vi "testpsp.vi"() -> ()   [LabVIEW 2013, in "testvarlib.lvlib"]
uses:
  testvarlib.lvlib
  execution/Scan Engine runtime.lvclass
  <vilib>/NI/Tag Bus Module Framework/channel/channel classification.ctl
  configuration/url prefix.ctl
  <vilib>/NI/Tag Bus/tag/Data Type.ctl
  configuration/Scan Engine configuration.lvclass
  configuration/Scan Engine configuration.lvclass/Scan Engine configuration.ctl
  <vilib>/NI/Tag Bus/table/data polymorphs/write one/write Double.vi
  <vilib>/NI/Tag Bus/table/data polymorphs/read one/read Double.vi
  configuration/Write discover channels.vi
  configuration/Write configure scan engine.vi
  <vilib>/NI/Tag Bus/table/data table.lvlib
  <vilib>/NI/Tag Bus/tag/tag descriptor.lvclass
  <vilib>/NI/Tag Bus Module Framework/channel/TBM channel.lvclass
panel:
  in  "testvarin":dbl
  out "testvarout":dbl
  in  "testvaroutTB":dbl
  in  "stop":bool
  out "ok":bool
  out "testvarinTB":dbl
  out "final error":errorcluster
  out "output error":errorcluster
  out "input error":errorcluster
  out "init error":errorcluster
  out "correct execution settings":bool
  out "serialization problem":errorcluster
  out "invalid configuration":errorcluster
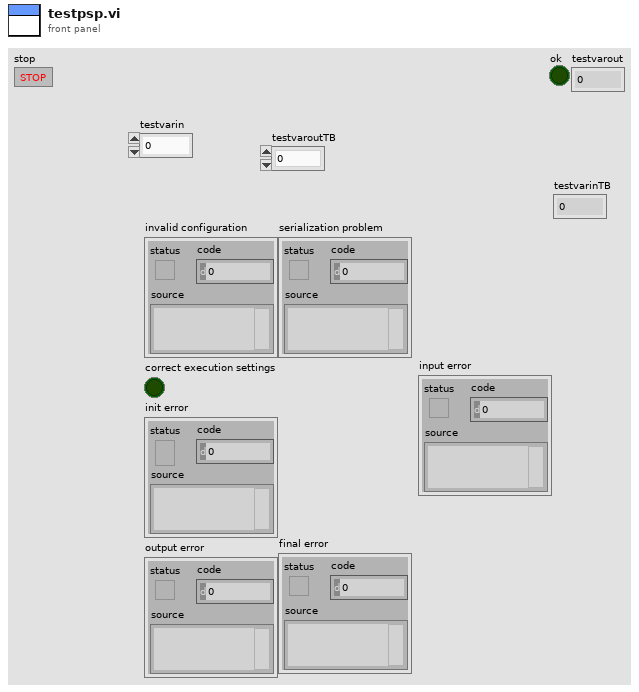
[diagram p1: front panel]
types:
  T1 = typedef "TBM channel.lvclass/channel classification.ctl" = enum16{"input data", "output data", "processing parameter", "processing result"}
  T2 = typedef "tag bus.lvlib/tag descriptor.lvclass/Data Type.ctl" = enum16{"Double", "Single", "I64", "I32", "I16", "I8", "U64", "U32", "U16", "U8", "Boolean", "String", "Array of Double", "Array of Single", "Array of I64", "Array of I32", "Array of I16", "Array of I8", "Array of U64", "Array of U32", "Array of U16", "Array of U8", "Array of Boolean", "Array of String"}
  T3 = typedef "Scan Engine configuration.lvclass/url prefix.ctl" = enum32{"ni.var.io://", "ni.var.psp://"}
  T4 = typedef "TBM channel.lvclass/data tables.ctl" = cluster{"input data":T5, "processing parameter":T5, "processing result":T5, "output data":T5}
  T5 = typedef "tag bus.lvlib/dictionary table pair.ctl" = cluster{"data dictionary":refnum<class "data dictionary.lvclass">, "data table":T6}
  T6 = typedef "tag bus.lvlib/data table.lvlib/data table.ctl" = cluster{"Double":dbl[], "Single":sgl[], "I64":i64[], "I32":i32[], "I16":i16[], "I8":i8[], "U64":u64[], "U32":u32[], "U16":u16[], "U8":u8[], "Boolean":bool[], "String":string[], "Array of Double":cluster{"DBL Array":dbl[]}[], "Array of Single":cluster{"SGL Array":sgl[]}[], "Array of I64":cluster{"I64 Array":i64[]}[], "Array of I32":cluster{"I32 Array":i32[]}[], "Array of I16":cluster{"I16 Array":i16[]}[], "Array of I8":cluster{"I8 Array":i8[]}[], "Array of U64":cluster{"U64 Array":u64[]}[], "Array of U32":cluster{"U32 Array":u32[]}[], "Array of U16":cluster{"U16 Array":u16[]}[], "Array of U8":cluster{"U8 Array":u8[]}[], "Array of Boolean":cluster{"Boolean Array":bool[]}[], "Array of String":cluster{"String Array":string[]}[]}
  T7 = typedef "TBM module execution interface.lvclass/execution settings.ctl" = cluster{"reads inputs":bool, "processes data":bool, "writes outputs":bool}
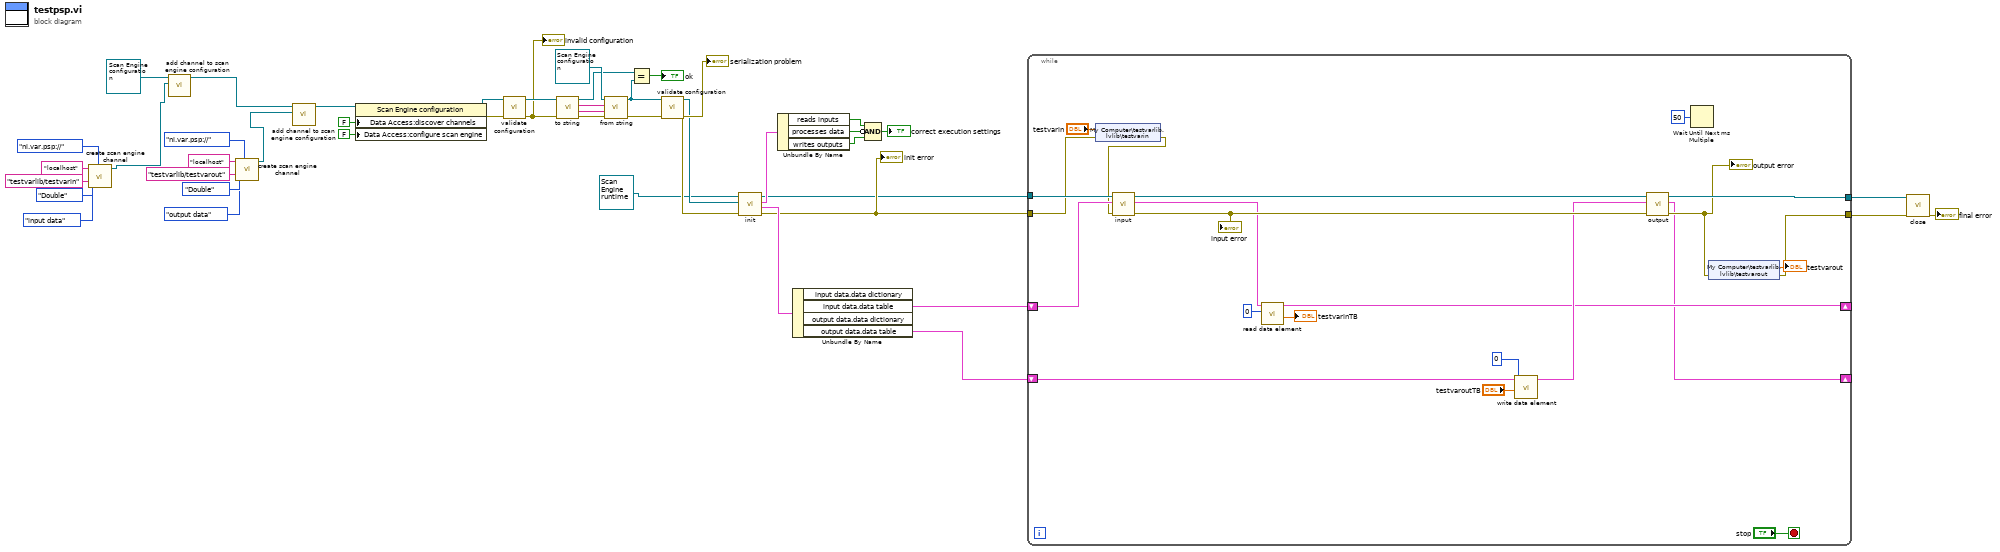
[diagram p0: block diagram]
diagram:
  n1 = call "create scan engine channel.vi"("URL"=url_prefix."ni.var.psp://", "channel classification"=channel_classification."input data", "data type"=Data_Type."Double", "variable name"="testvarlib/testvarin", "hostname"="localhost") -> ("channel"=w8:refnum<class "TBM channel.lvclass">)  [unwired: 6 in]
  n2 = call "add channel to scan engine configuration.vi"("channel"=w8, "Scan Engine configuration in"=refnum<class "Scan Engine configuration.lvclass"> refnum ("Scan Engine configuration")) -> ("Scan Engine configuration out"=w19:refnum<class "Scan Engine configuration.lvclass">)  [unwired: 8 in, 1 out]
  n3 = call "create scan engine channel.vi"("URL"=url_prefix."ni.var.psp://", "channel classification"=channel_classification."output data", "data type"=Data_Type."Double", "variable name"="testvarlib/testvarout", "hostname"="localhost") -> ("channel"=w7:refnum<class "TBM channel.lvclass">)  [unwired: 6 in]
  n4 = call "add channel to scan engine configuration.vi"("channel"=w7, "Scan Engine configuration in"=w19) -> ("Scan Engine configuration out"=w20:refnum<class "Scan Engine configuration.lvclass">)  [unwired: 8 in, 1 out]
  n5 = property class="Scan Engine configuration"(reference=w20, "Data Access:discover channels"=FALSE ("discover channels"), "Data Access:configure scan engine"=FALSE ("configure scan engine")) -> (reference out=w26:refnum<class "Scan Engine configuration.lvclass">, error out=w25:errorcluster)  [unwired: 1 in]
  n6 = call-dynamic "validate configuration.vi"("error in"=w25, "Scan Engine configuration in"=w26) -> ("error out"=w44:errorcluster, "Scan Engine configuration out"=w45:refnum<class "Scan Engine configuration.lvclass">)  [unwired: 8 in]
  "invalid configuration" <- w44
  n7 = call-dynamic "to string.vi"("error in"=w44, "Scan Engine configuration in"=w45) -> ("error out"=w41:errorcluster, "data"=w42:string, "version"=w43:string, "Scan Engine configuration out"=w4:refnum<class "Scan Engine configuration.lvclass">)  [unwired: 6 in]
  n8 = call-dynamic "from string.vi"("error in"=w41, "data"=w42, "version"=w43, "Scan Engine configuration in"=refnum<class "Scan Engine configuration.lvclass"> refnum ("Scan Engine configuration")) -> ("error out"=w40:errorcluster, "Scan Engine configuration out"=w3:refnum<class "Scan Engine configuration.lvclass">)  [unwired: 6 in]
  n9 = Equal?(x=w4, y=w3) -> (x = y?=→"ok":bool)
  n10 = call-dynamic "validate configuration.vi"("error in"=w40, "Scan Engine configuration in"=w3) -> ("error out"=w22:errorcluster, "Scan Engine configuration out"=w21:refnum<class "Scan Engine configuration.lvclass">)  [unwired: 8 in]
  "serialization problem" <- w22
  n11 = call-dynamic "init.vi"("error in"=w22, "TBM module configuration in"=w21, "Scan Engine runtime in"=refnum<class "Scan Engine runtime.lvclass"> refnum ("Scan Engine runtime")) -> ("error out"=w33:errorcluster, "data allocations"=w34:T4, "execution settings"=w39:T7, "Scan Engine runtime out"=w31:refnum<class "Scan Engine runtime.lvclass">)  [unwired: 5 in]
  "init error" <- w33
  n12 = Unbundle By Name(w39) -> ("reads inputs"=w36:bool, "processes data"=w38:bool, "writes outputs"=w37:bool)
  n13 = Unbundle By Name(w34) -> ("input data.data table"=w32:T6, "output data.data table"=w30:T6)  [unwired: 2 out]
  n14 = Compound Arithmetic op=AND(w36, invert w38, w37) -> (→"correct execution settings":bool)
  n15 = while {
    tunnel: w33 -> [w53]
    tunnel: w31 -> [w66]
    tunnel: [w61] -> w29
    tunnel: [w50] -> w28
    shift-right: [w47] -> _
    shift-left: w32 -> [w67]
    shift-right: [w46] -> _
    shift-left: w30 -> [w65]
    stop <- "stop" stop-if-true
    n16 = shared-variable "My Computer\\testvarlib.lvlib\\testvarin"("testvarin", error in=w53) -> (error out=w52:errorcluster)
    n17 = call-dynamic "input.vi"("error in"=w52, "data table in"=w67, "Scan Engine runtime in"=w66) -> ("error out"=w64:errorcluster, "data table out"=w60:T6, "Scan Engine runtime out"=w63:refnum<class "Scan Engine runtime.lvclass">)  [unwired: 6 in]
    "input error" <- w64
    n18 = call-poly <vilib>:"read data element.vi"("index"=0, "data table in"=w60) -> ("value"=→"testvarinTB":dbl, "data table out"=w47:T6)  [unwired: 8 in]
    n19 = call-poly <vilib>:"write data element.vi"("value"="testvaroutTB", "index"=0, "data table in"=w65) -> ("data table out"=w62:T6)  [unwired: 8 in]
    n20 = call-dynamic "output.vi"("error in"=w64, "data table in"=w62, "Scan Engine runtime in"=w63) -> ("error out"=w51:errorcluster, "data table out"=w46:T6, "Scan Engine runtime out"=w61:refnum<class "Scan Engine runtime.lvclass">)  [unwired: 6 in]
    "output error" <- w51
    n21 = Wait Until Next ms Multiple(millisecond multiple=u32 50) -> ()  [unwired: 1 out]
    n22 = shared-variable "My Computer\\testvarlib.lvlib\\testvarout"(error in=w51) -> (→"testvarout":dbl, error out=w50:errorcluster)
  }
  n23 = call-dynamic "close.vi"("error in"=w28, "Scan Engine runtime in"=w29) -> ("error out"=→"final error":errorcluster)  [unwired: 9 in]
